vi "Destroy.vi"(8 "Error In":errorcluster, 11 "Pixel In":refnum<class "Pixel.lvclass">) -> (0 "Error Out":errorcluster)   [LabVIEW 2019, in "Pixel.lvclass"]
uses:
  Pixel.lvclass
  Display Element/Display Element.lvclass
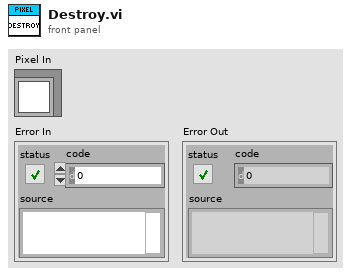
[diagram p1: front panel]
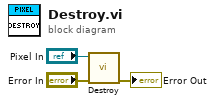
[diagram p0: block diagram]
diagram:
  n1 = call-parent "Destroy.vi"("Error In"="Error In", "Display Element In"="Pixel In") -> ("Error Out"=→"Error Out":errorcluster)  [unwired: 9 in]
